vi "ProcessImageHD_Poly.vi"   [LabVIEW 2022 SP3]
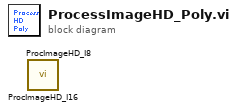
[diagram p0: block diagram]
diagram:
  n1 = call "ProcImageHD_I16.vi"() -> ()  [unwired: 8 in, 2 out]
  n2 = call "ProcImageHD_I8.vi"() -> ()  [unwired: 8 in, 2 out]
